vi "SaveMatrix.vi"(0 "Experiment Name":string, 1 "Identify Name":string, 2 "Data":dbl[][](array[numeric]), 3 "matrix_max":dbl, 4 "matrix_min":dbl, 5 "error in":errorcluster, 6 "File Name":string, 7 "Index Name":string, 8 "path":path, 10 "Specify Range?":bool=TRUE, 11 "Enable?":bool, 12 "Crop Pixels":u16=30, 13 "Time Stamp?":bool) -> (15 "img cancelled":bool, 19 "error out":errorcluster)   [LabVIEW 2018]
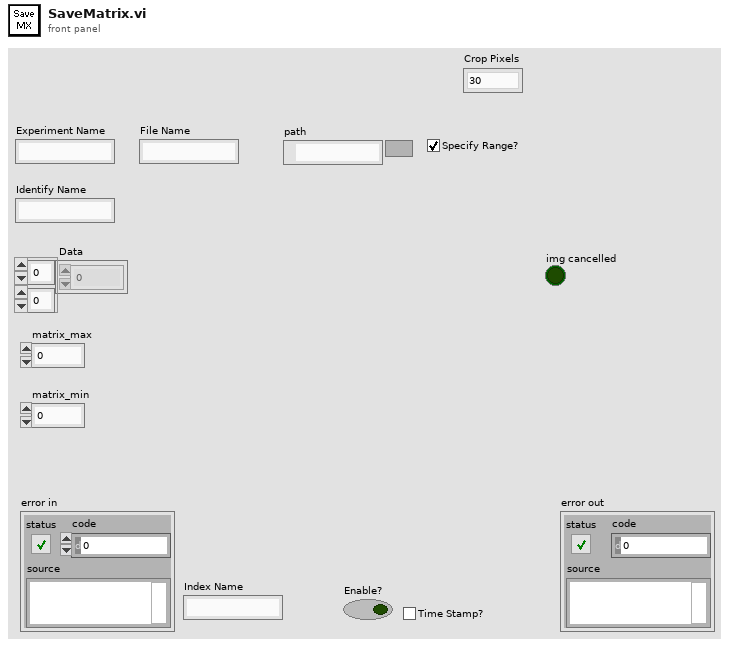
[diagram p1: front panel]
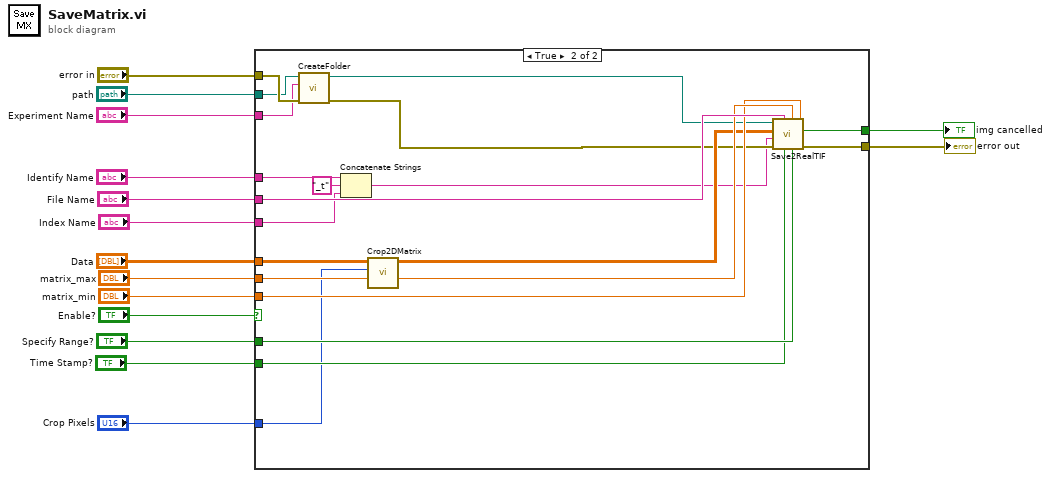
[diagram p0: block diagram]
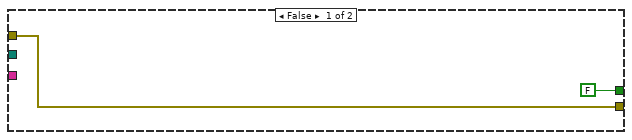
[diagram p2: hidden frame]
diagram:
  n1 = case shown="True" "Enable?" {
    tunnel: "error in" -> [w17 w26]
    tunnel: [w17 w36] -> w14
    tunnel: "Experiment Name" -> [_ w24]
    tunnel: "File Name" -> [_ w34]
    tunnel: "Data" -> [_ w29]
    tunnel: "path" -> [_ w25]
    tunnel: [FALSE ("save cancelled") w35] -> w5
    tunnel: "matrix_max" -> [_ w33]
    tunnel: "matrix_min" -> [_ w32]
    tunnel: "Identify Name" -> [_ w21]
    tunnel: "Time Stamp?" -> [_ w30]
    tunnel: "Specify Range?" -> [_ w31]
    tunnel: "Crop Pixels" -> [_ w27]
    tunnel: "Index Name" -> [_ w19]
    frame False {
    }
    frame True {
      n2 = call "CreateFolder.vi"("error in (no error)"=w26, "name"=w24, "base path"=w25) -> ("error out"=w22:errorcluster, "path out"=w23:path)  [unwired: 7 in]
      n3 = Concatenate Strings(w21, "_t" ("string"), w19) -> (w18:string)
      n4 = call "Crop2DMatrix.vi"("Crop Pixels"=w27, "Data"=w29) -> ("Cropped Data"=w28:dbl[][])  [unwired: 9 in]
      n5 = call "Save2RealTIF.vi"("min_value"=w32, "Specify Range?"=w31, "max_value"=w33, "Time Stamp?"=w30, "File Name Prefix"=w34, "error in"=w22, "Identify Name"=w18, "Data 2D Array"=w28, "Parent Directory"=w23) -> ("error out"=w36:errorcluster, "cancelled"=w35:bool)  [unwired: 1 in]
    }
  }
  "error out" <- w14
  "img cancelled" <- w5
